vi "Create.vi"(8 "error in":errorcluster, 11 "Device Profile in":refnum<class "Device Profile.lvclass">) -> (0 "error out":errorcluster, 3 "Device Profile out":refnum<class "Device Profile.lvclass">)   [LabVIEW 2020, in "CANopen.lvlib" / "Device Profile.lvclass"]
uses:
  Device Profile.lvclass
  Device Profile.lvclass/Device Profile.ctl
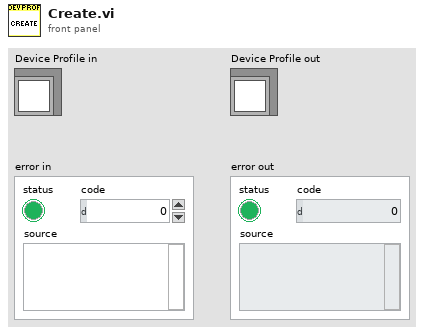
[diagram p1: front panel]
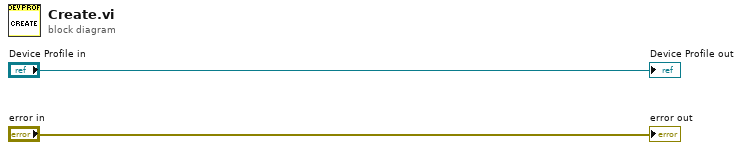
[diagram p0: block diagram]
diagram:
  "Device Profile out" <- "Device Profile in"
  "error out" <- "error in"
